vi "Write TempCoeff.vi"(8 "error in (no error)":errorcluster, 11 "BMP208 in":refnum<class "BMP208.lvclass">) -> (0 "error out":errorcluster, 3 "BMP208 out":refnum<class "BMP208.lvclass">)   [LabVIEW 2020, in "BMP208.lvclass"]
uses:
  BMP208.lvclass
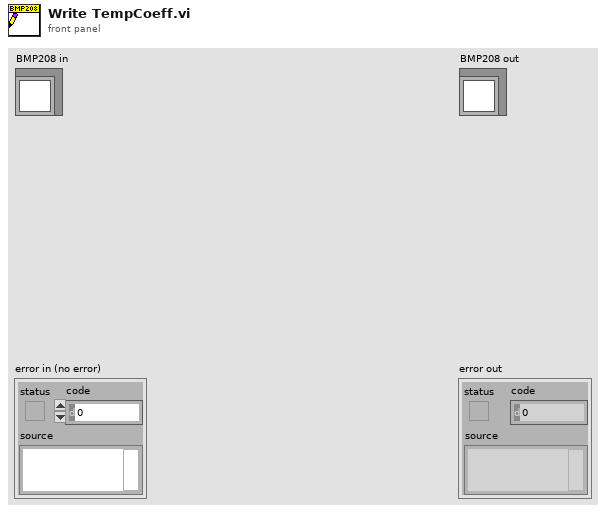
[diagram p1: front panel]
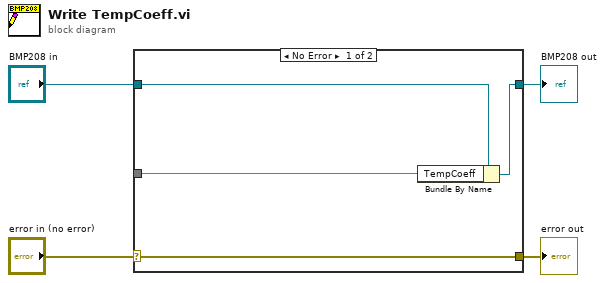
[diagram p0: block diagram]
diagram:
  n1 = case shown="No Error" "error in (no error)" {
    selector: "error in (no error)" -> [w8 w9]
    tunnel: [w8 w9] -> w3
    tunnel: [w6 w10] -> w1
    tunnel: "BMP208 in" -> [w7 w10]
    tunnel: _ -> [w5 _]
    frame No Error {
      n2 = Bundle By Name(cluster=w7, "TempCoeff"=w5) -> (w6:refnum<class "BMP208.lvclass">)
    }
    frame Error {
    }
  }
  "error out" <- w3
  "BMP208 out" <- w1
